vi "replaceBalanceToken.vi"(8 "error in (no error)":errorcluster, 10 "Query In":string, 11 "Transaction in":refnum<class "Transaction.lvclass">) -> (0 "error out":errorcluster, 2 "Query Out":string, 3 "Transaction out":refnum<class "Transaction.lvclass">)   [LabVIEW 2018, in "Transaction.lvclass"]
uses:
  Transaction.lvclass
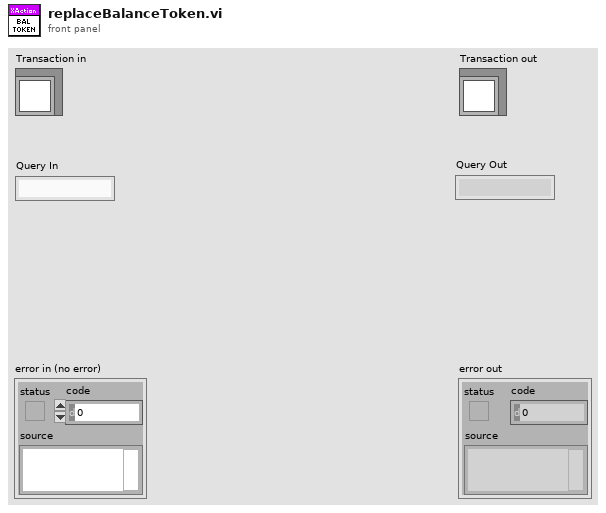
[diagram p1: front panel]
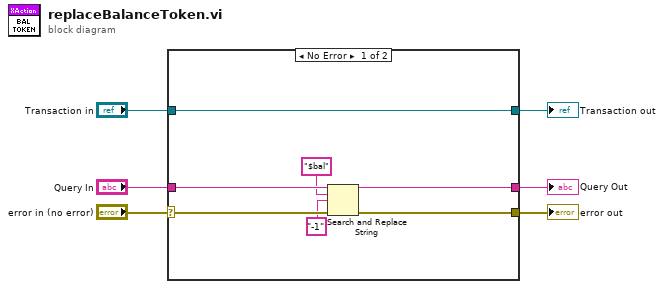
[diagram p0: block diagram]
diagram:
  n1 = case shown="No Error" "error in (no error)" {
    selector: "error in (no error)" -> [w10 w16]
    tunnel: [w9 w16] -> w5
    tunnel: [w13 w15] -> w3
    tunnel: "Transaction in" -> [w13 w15]
    tunnel: "Query In" -> [w12 w14]
    tunnel: [w11 w14] -> w1
    frame No Error {
      n2 = Search and Replace String(input string=w12, search string="$bal", replace string="-1" ("replace string (\"\")"), error in=w10) -> (result string=w11:string, error out=w9:errorcluster)  [unwired: 4 in, 2 out]
    }
    frame Error {
    }
  }
  "error out" <- w5
  "Transaction out" <- w3
  "Query Out" <- w1
